vi "Problem 21.vi"(11 "Limit":i32) -> (2 "Amicable Numbers":i32[](array[numeric]), 3 "Sum of Amicable #s":i32)   [LabVIEW 2013, in "Problem 21.lvlib"]
uses:
  Problem 21.lvlib
  <userlib>/_OpenG.lib/array/array.llb/Remove Duplicates from 1D Array (I32)__ogtk.vi
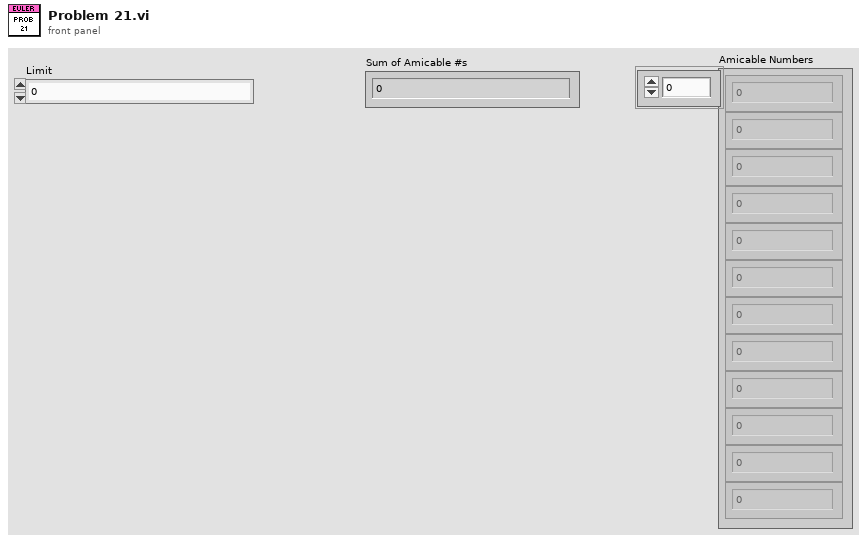
[diagram p1: front panel]
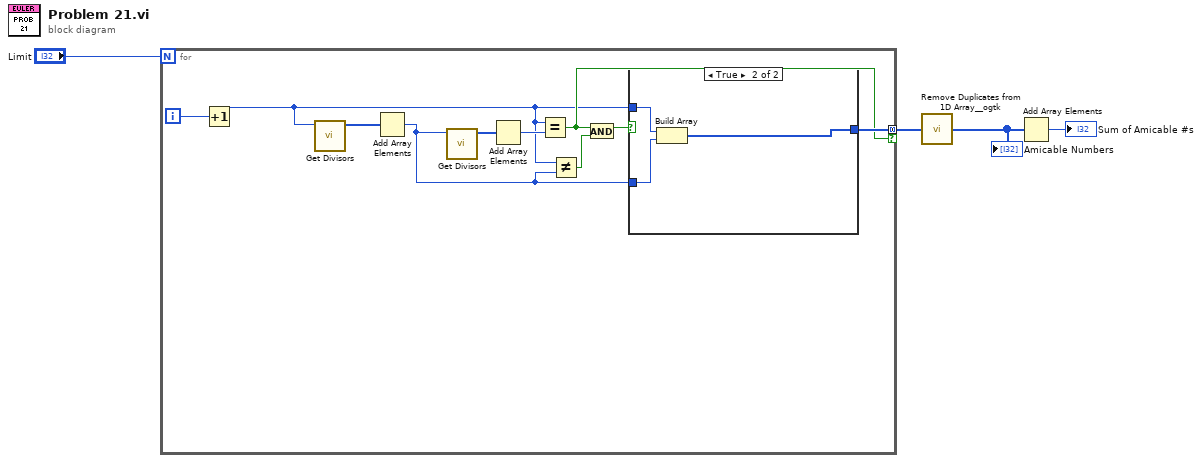
[diagram p0: block diagram]
diagram:
  n1 = for {
    N: "Limit" -> [_]
    tunnel: [w12] -> w3 mode=concatenating if=w11
    i -> [w14]
    n2 = Increment(x=w14) -> (x+1=w6:i32)
    n3 = call "Get Divisors.vi"("Number"=w6) -> ("Divisors"=w10:i32[])  [unwired: 10 in]
    n4 = Add Array Elements(numeric array=w10) -> (sum=w5:i32)
    n5 = call "Get Divisors.vi"("Number"=w5) -> ("Divisors"=w9:i32[])  [unwired: 10 in]
    n6 = Add Array Elements(numeric array=w9) -> (sum=w13:i32)
    n7 = Equal?(x=w6, y=w13) -> (x = y?=w11:bool)
    n8 = Not Equal?(x=w6, y=w5) -> (x != y?=w7:bool)
    n9 = And(x=w11, y=w7) -> (x .and. y?=w8:bool)
    n10 = case shown="True" w8 {
      tunnel: w5 -> [_ w16]
      tunnel: w6 -> [_ w17]
      tunnel: [_ w15] -> w12
      frame False {
      }
      frame True {
        n11 = Build Array(w17, w16) -> (w15:i32[])
      }
    }
  }
  n12 = call-poly <userlib>:"Remove Duplicates from 1D Array__ogtk.vi"("Input Array"=w3) -> ("Output Array"=w1:i32[])  [unwired: 1 out]
  "Amicable Numbers" <- w1
  n13 = Add Array Elements(numeric array=w1) -> (sum=→"Sum of Amicable #s":i32)
